vi "Encoder to Turret.vi"(11 "Encoder":dbl) -> (3 "Turret Angle":dbl)   [LabVIEW 2019]
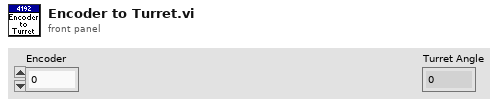
[diagram p1: front panel]
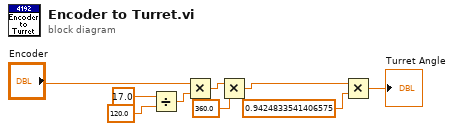
[diagram p0: block diagram]
diagram:
  n1 = Divide(x=17.0, y=120.0) -> (x/y=w7:dbl)
  n2 = Multiply(x="Encoder", y=w7) -> (x*y=w6:dbl)
  n3 = Multiply(x=w6, y=360.0) -> (x*y=w4:dbl)
  n4 = Multiply(x=w4, y=0.9424833541406575) -> (x*y=→"Turret Angle":dbl)
